vi "Adjusted_Rand_Score.vi"(8 "error in":errorcluster caption="entrée d'erreur", 10 "labels_pred":string[][](array[string]), 11 "labels_true":string[][](array[string])) -> (0 "error out":errorcluster caption="sortie d'erreur", 3 "Score":string)   [LabVIEW 2020]
doc: "Rand index adjusted for chance.\n\nThe Rand Index computes a similarity measure between two clusterings by considering all pairs of samples and counting pairs that are assigned in the same or different clusters in the predicted and true clusterings.\n\nThe raw RI score is then “adjusted for chance” into the ARI score using the following scheme:\n\nARI = (RI - Expected_RI) / (max(RI) - Expected_RI)\n\nThe adjusted Rand index is thus ensured to have a value close to 0.0 for random labeling independently of the number of clusters and samples and exactly 1.0 when the clusterings are identical (up to a permutation).\n\nARI is a symmetric measure :\n\nadjusted_rand_score(a, b) == adjusted_rand_score(b, a)\n\n\nParameters :\n\n- labels_true : int array, shape = [n_samples]\nGround truth class labels to be used as a reference\n\n- labels_pred : array-like of shape (n_samples,)\nCluster labels to evaluate\n\nReturns : \n\n- ari : float\nSimilarity score between -1.0 and 1.0. Random labelings have an ARI close to 0.0. 1.0 stands for perfect match."
uses:
  Adjusted_Rand_Score.lvclass
panel:
  out "Adjusted_Rand_Score.lvclass":refnum<class "Adjusted_Rand_Score.lvclass">
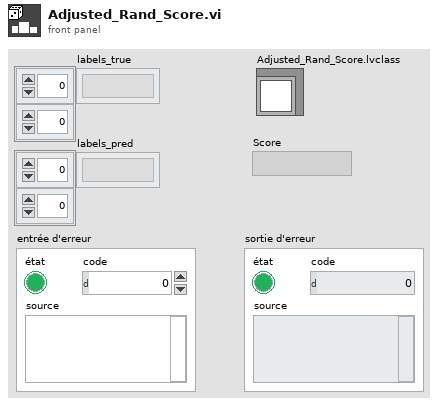
[diagram p1: front panel]
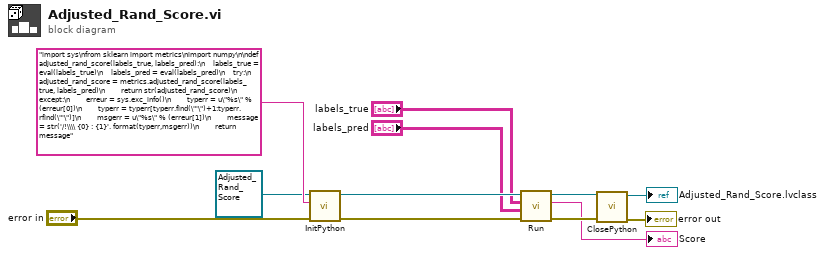
[diagram p0: block diagram]
diagram:
  n1 = call-dynamic "InitPython.vi"("error in (no error)"="error in", "Python Instruction"="import sys\nfrom sklearn import metrics\nimport numpy\n\ndef adjusted_rand_score(labels_true, labels_pred):\n    labels_true = eval(labels_true)\n    labels_pred = eval(labels_pred)\n    try:\n        adjusted_rand_score = metrics.adjusted_rand_score(labels_true, labels_pred)\n        return str(adjusted_rand_score)\n    except:\n        erreur = sys.exc_info()\n        typerr = u\"%s\" % (erreur[0])\n        typerr = typerr[typerr.find(\"'\")+1:typerr.rfind(\"'\")]\n        msgerr = u\"%s\" % (erreur[1])\n        message = str('/!\\\\ {0} : {1}'. format(typerr,msgerr))\n        return message", "Scikit-learn en entrée"=refnum<class "Adjusted_Rand_Score.lvclass"> refnum ("Adjusted_Rand_Score.lvclass")) -> ("error out"=w7:errorcluster, "Scikit-learn en sortie"=w8:refnum<class "Adjusted_Rand_Score.lvclass">)  [unwired: 7 in]
  n2 = call-dynamic "Run.vi"("error in (no error)"=w7, "labels_pred"="labels_pred", "labels_true"="labels_true", "Adjusted_Rand_Score.lvclass"=w8) -> ("error out"=w5:errorcluster, "String Data"=→"Score":string, "Adjusted_Rand_Score.lvclass"=w6:refnum<class "Adjusted_Rand_Score.lvclass">)  [unwired: 5 in]
  n3 = call-dynamic "ClosePython.vi"("error in (no error)"=w5, "Scikit-learn en entrée"=w6) -> ("error out"=→"error out":errorcluster, "Scikit-learn en sortie"=→"Adjusted_Rand_Score.lvclass":refnum<class "Adjusted_Rand_Score.lvclass">)  [unwired: 8 in]
